vi "SAlabView.vi"() -> ()   [LabVIEW 2022 SP3]
uses:
  riversideSAFilter.dll
panel:
  in  "downfactor":u16
  out "min value 2":i16
  out "max value":i16
  out "min value":i16
  out "duration (ms)":u32
  in  "Filter Prams":T1={"low cutoff"=20, "order"=51, "high cutoff"=55}
  in  "filter type":T2(ring)=enum."Bandpass"
  in  "selected path 2":path=path "E:/LabVIEW 2016 Suite/GPU_HK/LabVIEW Example/riversideTdrGeometry.bin"
  in  "selected path":path=path "E:/LabVIEW 2016 Suite/GPU_HK/LabVIEW Example/eyeData.bin"
  in  "time start [s]":sgl[](array[numeric])=[8.754e-06, 8.754e-06, 8.754e-06, 8.754e-06, 8.754e-06, 8.754e-06, 8.754e-06, 8.754e-06, 8.754e-06, 8.754e-06, 8.754e-06, 8.754e-06, 8.754e-06, 8.754e-06, 8.754e-06, 8.754e-06, 8.754e-06, 8.754e-06, 8.754e-06, 8.754e-06, 8.754e-06, 8.754e-06, 8.754e-06, 8.754e-06, 8.754e-06, 1.0, 1.0, 1.0, 1.0, 1.0, 1.0, 1.0, 1.0, 1.0, 1.0, 1.0, 1.0, 1.0, 1.0, 1.0, 1.0, 1.0, 1.0, 1.0, 1.0, 1.0, 1.0, 1.0, 1.0, 1.0]
  in  "weighting":sgl[](array[numeric])=[1.0, 1.0, 1.0, 1.0, 1.0, 1.0, 1.0, 1.0, 1.0, 1.0, 1.0, 1.0, 1.0, 1.0, 1.0, 1.0, 1.0, 1.0, 1.0, 1.0, 1.0, 1.0, 1.0, 1.0, 1.0, 1.0, 1.0, 1.0, 1.0, 1.0, 1.0, 1.0, 1.0, 1.0, 1.0, 1.0, 1.0, 1.0, 1.0, 1.0, 1.0, 1.0, 1.0, 1.0, 1.0, 1.0, 1.0, 1.0, 1.0, 1.0]
  in  "Number of Tx/Rx pair":i32=25
  in  "Receive Element #":i32[](array[numeric])=[0, 1, 2, 3, 4, 0, 1, 2, 3, 4, 0, 1, 2, 3, 4, 0, 1, 2, 3, 4, 0, 1, 2, 3, 4, 0, 1, 2, 3, 4, 0, 1, 2, 3, 4, 0, 1, 2, 3, 4, 0, 1, 2, 3, 4, 0, 1, 2, 3, 4]
  in  "Tramsmit Element #":i32[](array[numeric])=[0, 0, 0, 0, 0, 1, 1, 1, 1, 1, 2, 2, 2, 2, 2, 3, 3, 3, 3, 3, 4, 4, 4, 4, 4, 0, 0, 0, 0, 0, 1, 1, 1, 1, 1, 2, 2, 2, 2, 2, 3, 3, 3, 3, 3, 4, 4, 4, 4, 4]
  in  "Speed of sound [m/s]":i32=1540
  out "data from file 2":sgl[](graph)
  out "Log B-mode image":dbl[][](graph)
  in  "Number of channel":i32=5
  in  "Number of received sample per scanline":i32=3500
  in  "Number of scanline":i32=201
  out "data from file":i8[](graph)
  in  "Sampling Frequency [MHz]":i32=250
  out "nError":i32
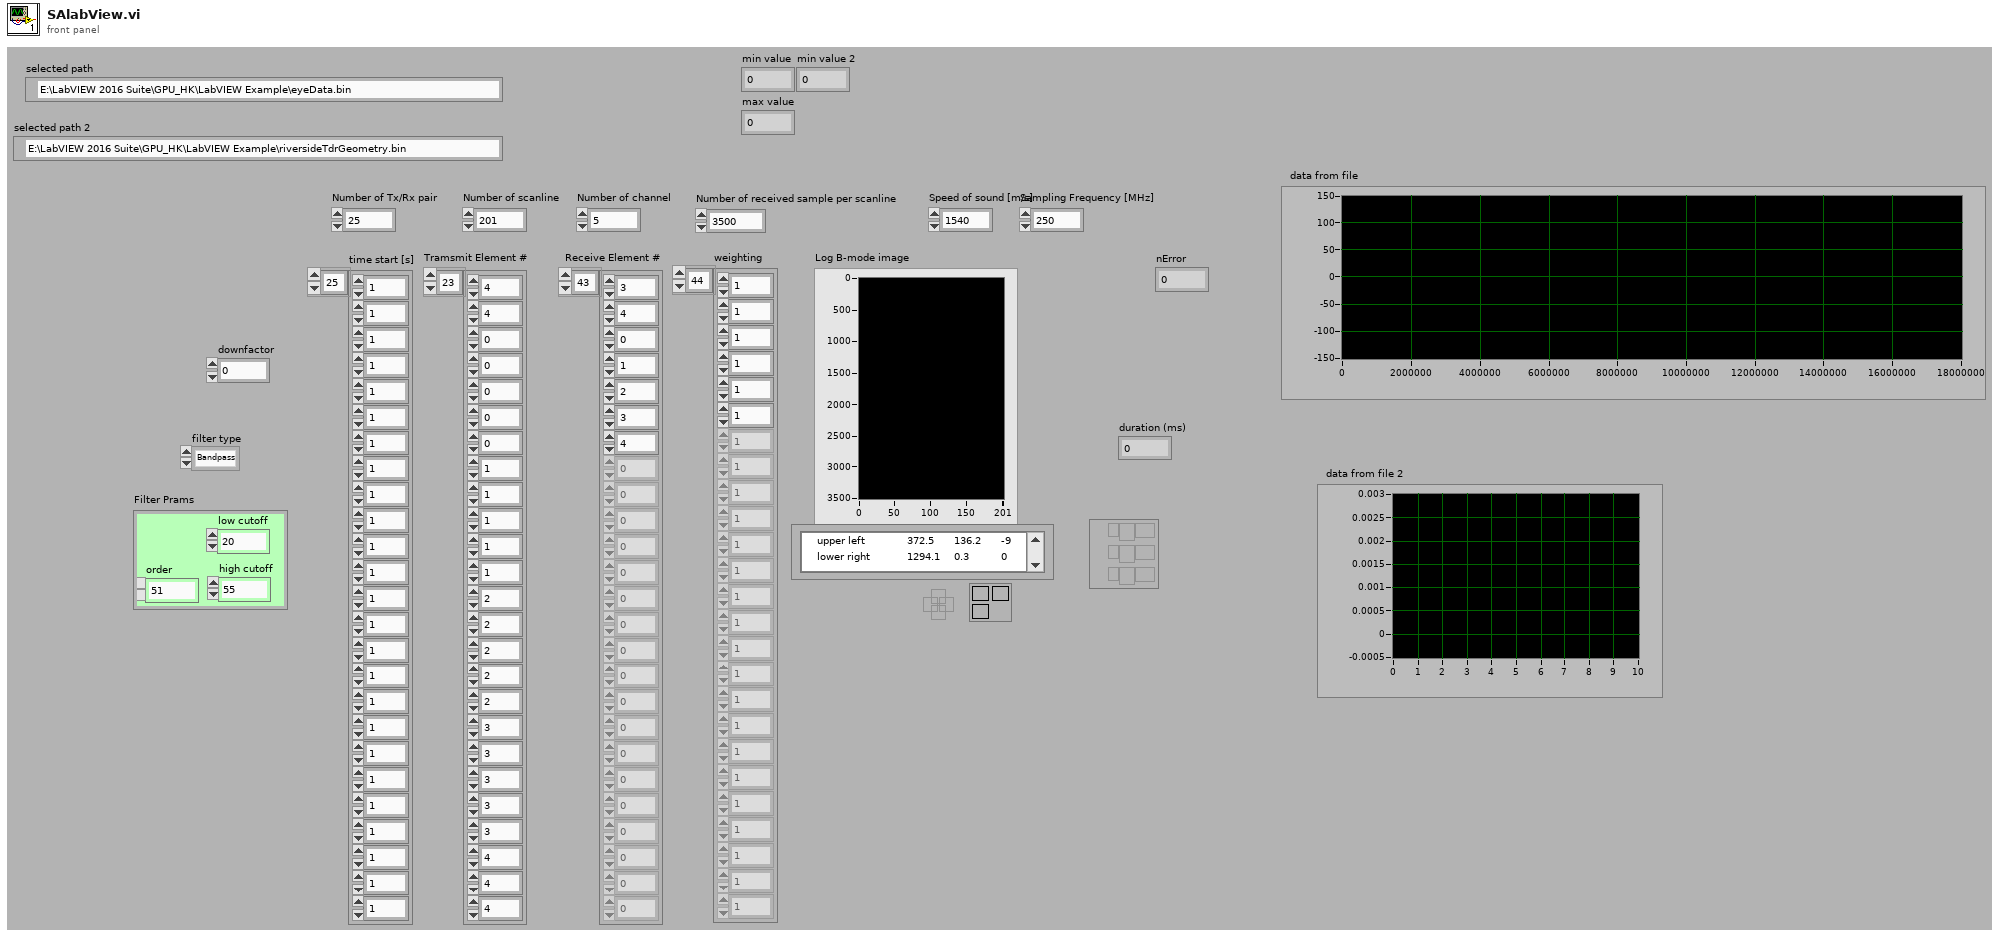
[diagram p1: front panel]
types:
  T1 = cluster{"low cutoff":i32, "order":i32, "high cutoff":i32}
  T2 = enum32{"Lowpass", "Highpass", "Bandpass", "Bandstop"}
  T3 = enum16{"open", "replace", "create", "open or create", "replace or create", "replace or create with confirmation"}
  T4 = enum16{"deny read/write", "deny write-only", "deny none"}
  T5 = enum16{"big-endian, network order", "native, host order", "little-endian"}
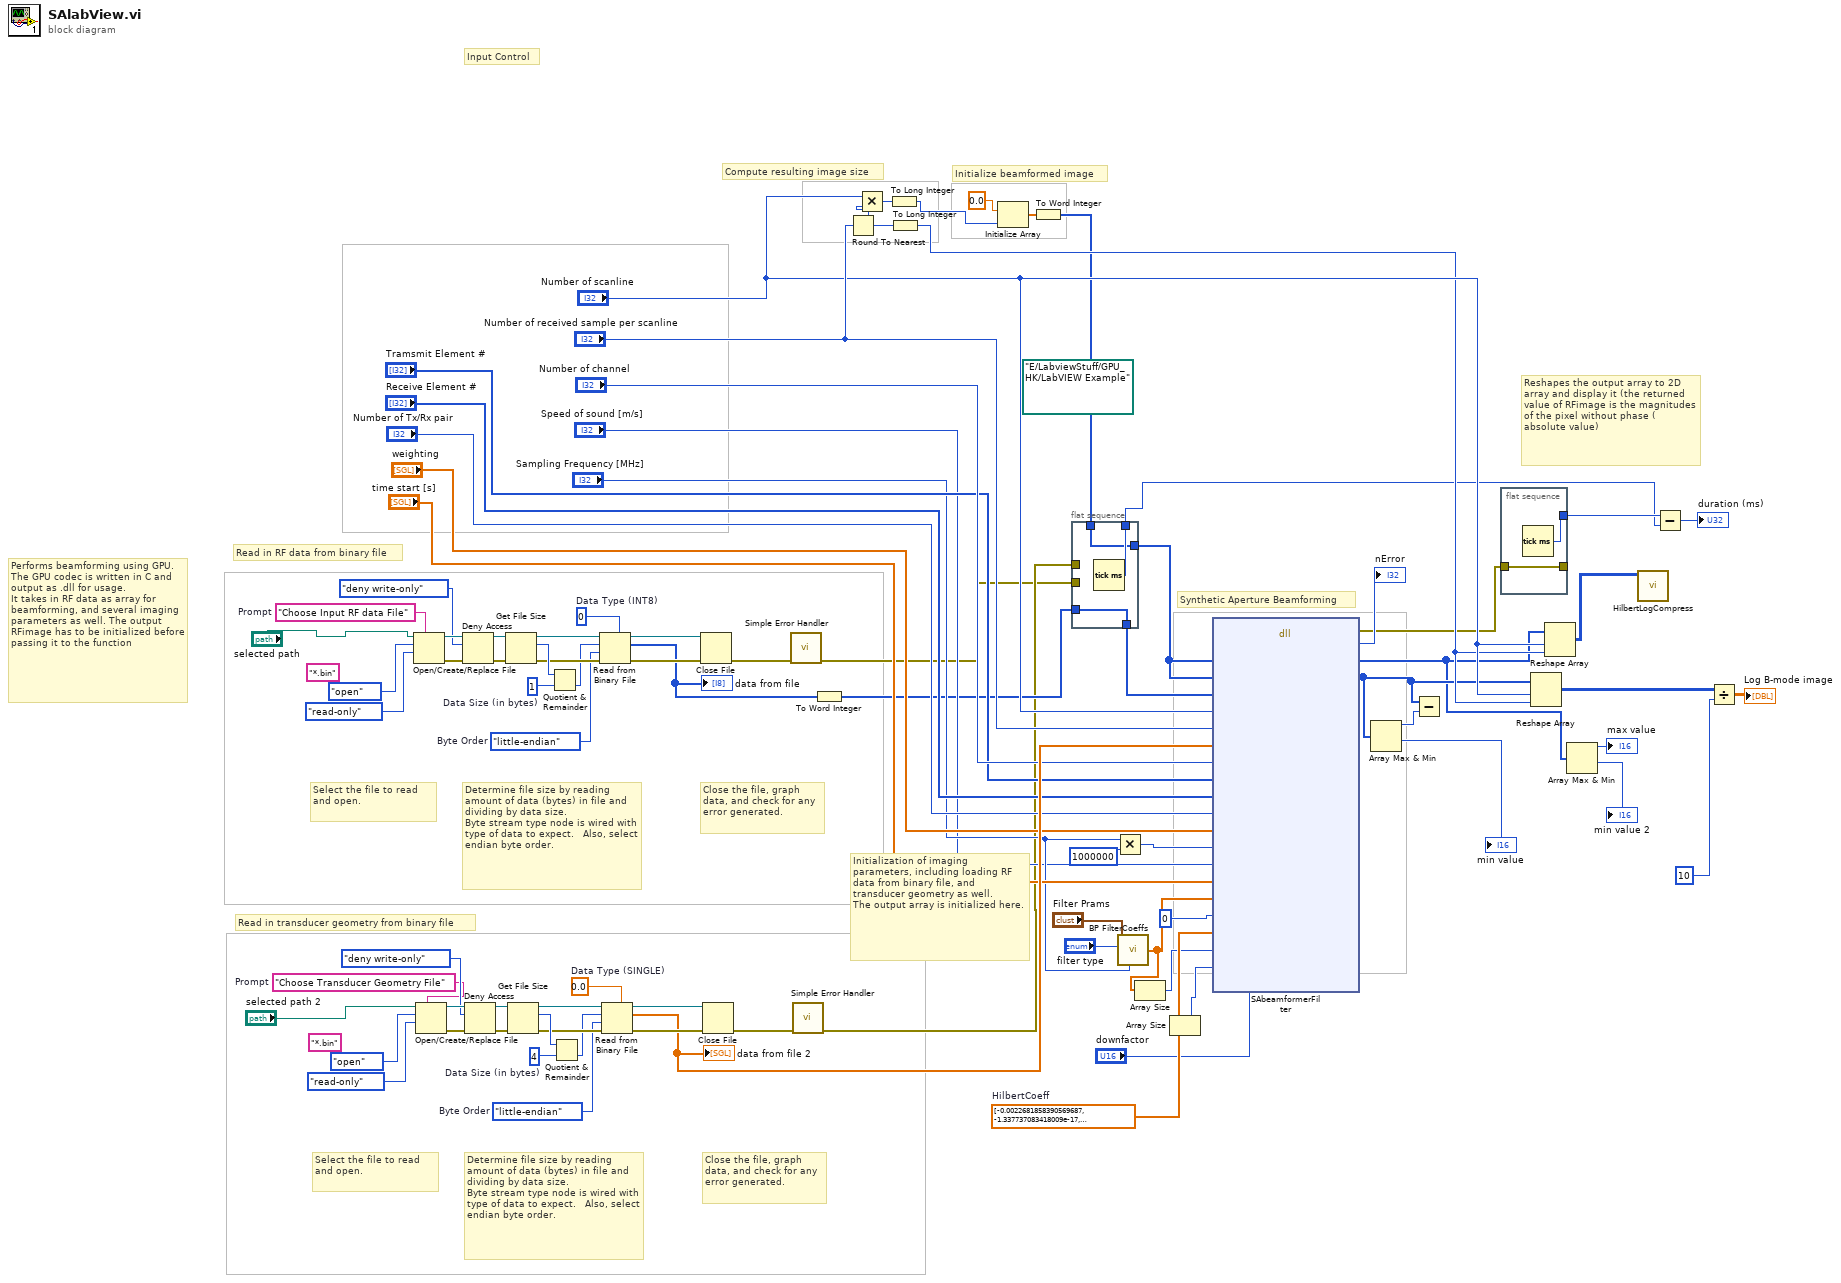
[diagram p0: block diagram]
diagram:
  w14 = sgl[] [-0.0022681858, -1.3377371e-17, -0.0041749156, 1.3026156e-17, -0.0068346895, -4.195826e-17, -0.010427003, -1.1244341e-16, -0.015182828, -3.725316e-17, -0.021423787, -1.1259981e-16, -0.029640518, -9.678795e-17, -0.040659484, -5.638797e-17, -0.05603469, 9.1425055e-18, -0.079112425, -9.958648e-17, -0.118650794, 1.000237e-18, -0.20691232, -6.3757414e-17, -0.6348398, 0.0, 0.6348398, 6.3757414e-17, 0.20691232, -1.000237e-18, 0.118650794, 9.958648e-17, 0.079112425, -9.1425055e-18, 0.05603469, 5.638797e-17, 0.040659484, 9.678795e-17, 0.029640518, 1.1259981e-16, 0.021423787, 3.725316e-17, 0.015182828, 1.1244341e-16, 0.010427003, 4.195826e-17, 0.0068346895, -1.3026156e-17, 0.0041749156, 1.3377371e-17, 0.0022681858]  # HilbertCoeff
  (unwired) path "E:/LabviewStuff/GPU_HK/LabVIEW Example" ("Set Directory")
  w57 = T5."little-endian"  # Byte Order
  w59 = i64 4  # Data Size (in bytes)
  w60 = sgl 0.0  # Data Type (SINGLE)
  (unwired) "*.bin" ("pattern (all files)")
  w34 = "Choose Transducer Geometry File"  # Prompt
  w76 = T5."little-endian"  # Byte Order
  w78 = i64 1  # Data Size (in bytes)
  w79 = i8 0  # Data Type (INT8)
  (unwired) "*.bin" ("pattern (all files)")
  w36 = "Choose Input RF data File"  # Prompt
  # "Reshapes the output array to 2D array and display it (the returned value of RFimage is the magnitudes of the pixel without phase ( absolute value)"
  # "Performs beamforming using GPU. The GPU codec is written in C and output as .dll for usage.\nIt takes in RF data as array for beamforming, and several imaging parameters as well. The output RFimage has to be initialized before passing it to the function"
  # "Initialization of imaging parameters, including loading RF data from binary file, and transducer geometry as well.\nThe output array is initialized here."
  # "Read in transducer geometry from binary file"
  # "Close the file, graph data, and check for any error generated."
  # "Determine file size by reading amount of data (bytes) in file and dividing by data size.\nByte stream type node is wired with\ntype of data to expect.   Also, select endian byte order."
  # "Select the file to read and open."
  # "Compute resulting image size"
  # "Initialize beamformed image"
  # "Synthetic Aperture Beamforming"
  # "Input Control"
  # "Read in RF data from binary file"
  # "Close the file, graph data, and check for any error generated."
  # "Determine file size by reading amount of data (bytes) in file and dividing by data size.\nByte stream type node is wired with\ntype of data to expect.   Also, select endian byte order."
  # "Select the file to read and open."
  n1 = Open/Create/Replace File(file path (use dialog)="selected path", prompt=w36, operation (0:open)=T3."open", access (0:read/write)=enum16{"read/write", "read-only", "write-only"}."read-only") -> (refnum out=w74:refnum<file>, error out=w75:errorcluster)  [unwired: 2 in, 1 out]
  n2 = Open/Create/Replace File(file path (use dialog)="selected path 2", prompt=w34, operation (0:open)=T3."open", access (0:read/write)=enum16{"read/write", "read-only", "write-only"}."read-only") -> (refnum out=w55:refnum<file>, error out=w56:errorcluster)  [unwired: 2 in, 1 out]
  n3 = Deny Access(4:w75, 6:T4."deny write-only" ("deny mode (0:deny read/write)"), 7:w74) -> (0:w73:errorcluster, 3:w72:refnum<file>)
  n4 = Deny Access(4:w56, 6:T4."deny write-only" ("deny mode (0:deny read/write)"), 7:w55) -> (0:w54:errorcluster, 3:w53:refnum<file>)
  n5 = Get File Size(file=w72, error in=w73) -> (refnum out=w86:refnum<file>, size (in bytes)=w82:i64, 0:w81:errorcluster)
  n6 = Get File Size(file=w53, error in=w54) -> (refnum out=w67:refnum<file>, size (in bytes)=w63:i64, 0:w62:errorcluster)
  n7 = Quotient & Remainder(x=w82, y=w78) -> (floor(x/y)=w77:i64)  [unwired: 1 out]
  n8 = Quotient & Remainder(x=w63, y=w59) -> (floor(x/y)=w58:i64)  [unwired: 1 out]
  n9 = Read from Binary File(5:w79, 8:w81, 9:w76, 10:w77, 11:w86) -> (0:w84:errorcluster, 2:w37:i8[], 3:w85:refnum<file>)  [unwired: 1 in, 1 out]
  "data from file" <- w37
  n10 = Read from Binary File(5:w60, 8:w62, 9:w57, 10:w58, 11:w67) -> (0:w65:errorcluster, 2:w47:sgl[], 3:w66:refnum<file>)  [unwired: 1 in, 1 out]
  "data from file 2" <- w47
  n11 = Close File(refnum=w85, error in=w84) -> (error out=w83:errorcluster)  [unwired: 1 out]
  n12 = Close File(refnum=w66, error in=w65) -> (error out=w64:errorcluster)  [unwired: 1 out]
  n13 = call <vilib>:"Simple Error Handler.vi"("error in (no error)"=w83) -> ("error out"=w18:errorcluster)  [unwired: 4 in, 4 out]
  n14 = call <vilib>:"Simple Error Handler.vi"("error in (no error)"=w64) -> ("error out"=w19:errorcluster)  [unwired: 4 in, 4 out]
  n15 = To Word Integer(number=w37) -> (16bit integer=w21:i16[])
  n16 = Round To Nearest(number="Number of received sample per scanline") -> (nearest integer value=w39:i32)
  n17 = Multiply(x="Number of scanline", y=w39) -> (x*y=w68:i32)
  n18 = To Long Integer(number=w68) -> (32bit integer=w50:i32)
  n19 = To Long Integer(number=w39) -> (32bit integer=w28:i32)
  n20 = Initialize Array(0.0 ("element"), w50) -> (w69:dbl[])
  n21 = To Word Integer(number=w69) -> (16bit integer=w17:i16[])
  n22 = flat-sequence {
    tunnel: [w90] -> w23
    tunnel: w21 -> [w89]
    tunnel: [w89] -> w20
    tunnel: w19 -> [_]
    tunnel: w18 -> [_]
    tunnel: w17 -> [w88]
    tunnel: [w88] -> w16
    frame #0 {
      n23 = Tick Count (ms)() -> (millisecond timer value=w90:u32)
    }
  }
  n24 = Multiply(x="Sampling Frequency [MHz]", y=1000000) -> (x*y=w40:i32)
  n25 = call "BP FilterCoeffs.vi"("sample rate MHz"="Sampling Frequency [MHz]", "Filter Prams"="Filter Prams", "filter type"="filter type") -> ("FIR Windowed Coefficients"=w13:dbl[])  [unwired: 3 in]
  n26 = Array Size(array=w13) -> (size(s)=w12:i32)
  n27 = Array Size(array=w14) -> (size(s)=w11:i32)
  n28 = dll-call lib="D:/LabVIEWSuite_64_OS/GPU_HK/LabVIEW Example/riversideSAFilter.dll" fn="SAbeamformerFilter"("RF_Out"=w16, "RFimage"=w16, "RFdata"=w20, "numScanline"="Number of scanline", "dataVectorLength"="Number of received sample per scanline", "TdrGeometry"=w47, "numChannel"="Number of channel", "txPos"="Tramsmit Element #", "rxPos"="Receive Element #", "numTxRxPair"="Number of Tx/Rx pair", "weighting"="weighting", "fs"=w40, "sos"="Speed of sound [m/s]", "time_start"="time start [s]", "BPfilter"=w13, "DataFlag"=0, "filter"=w14, "BPFILTERLENGTH"=w12, "FILTERLENGTH"=w11, "downfactor"="downfactor") -> (error out=w25:errorcluster, "nError"=→"nError":i32, "RF_Out"=w8:i16[], "RFimage"=w10:i16[])  [unwired: 21 in, 1 out]
  n29 = Array Max & Min(array=w10) -> (max value=w15:i16, min value=→"min value":i16)  [unwired: 2 out]
  n30 = Subtract(x=w10, y=w15) -> ()  [unwired: 1 out]
  n31 = flat-sequence {
    tunnel: w25 -> [w92]
    tunnel: [w92] -> _
    tunnel: [w91] -> w24
    frame #0 {
      n32 = Tick Count (ms)() -> (millisecond timer value=w91:u32)
    }
  }
  n33 = Reshape Array(w10, "Number of scanline", w28) -> (w2:i16[][])
  n34 = Reshape Array(w8, "Number of scanline", w28) -> (w5:i16[][])
  n35 = Array Max & Min(array=w8) -> (max value=→"max value":i16, min value=→"min value 2":i16)  [unwired: 2 out]
  n36 = call "HilbertLogCompress.vi"("Array in"=w5) -> ()  [unwired: 10 in, 1 out]
  n37 = Subtract(x=w24, y=w23) -> (x-y=→"duration (ms)":u32)
  n38 = Divide(x=w2, y=10) -> (x/y=→"Log B-mode image":dbl[][])
